vi "Serials.vi"() -> ()   [LabVIEW 2012]
panel:
  in  "ICImagingControl":refnum<k7>(container)
  out "Modelnames (hidden)":string[](array[string])
  out "Model Name":string
  out "Serials (hidden)":string[](array[string])
  in  "End Program":bool
  in  "Open & Snap":bool
  out "Serial":string
  in  "Devices":i32(listbox)
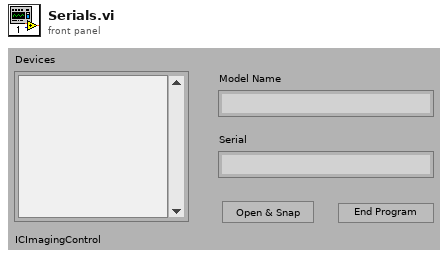
[diagram p1: front panel]
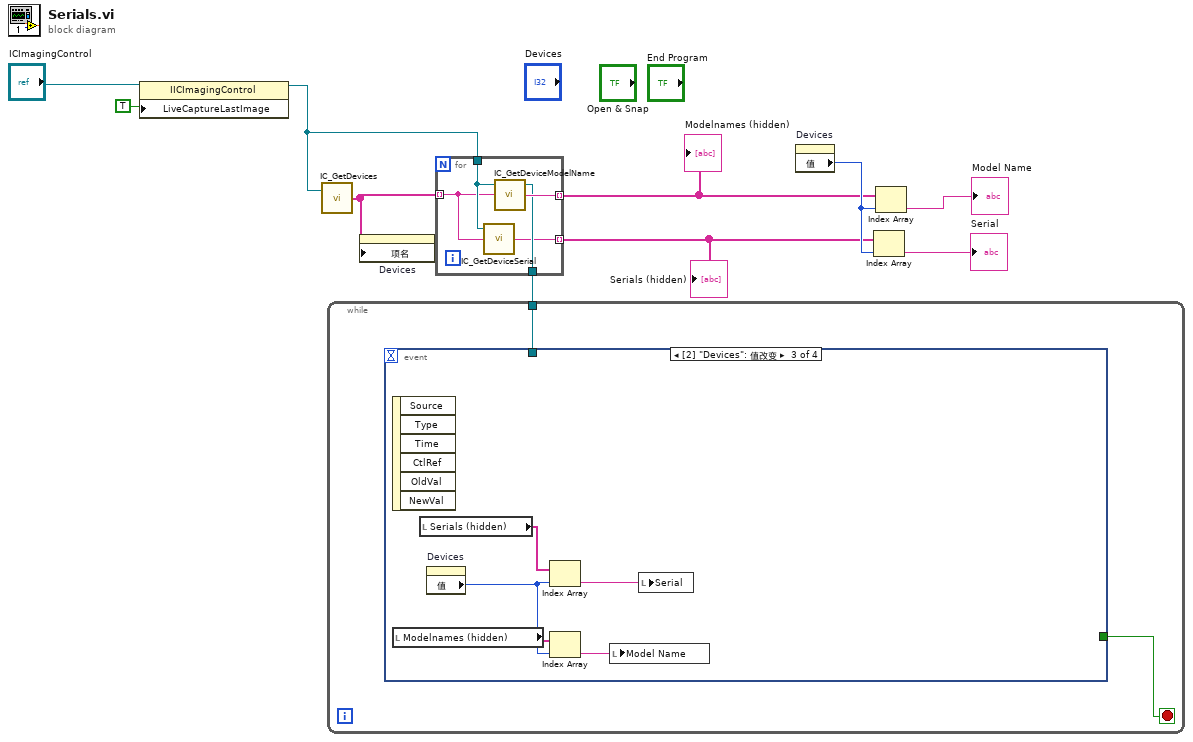
[diagram p0: block diagram]
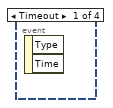
[diagram p2: hidden frame]
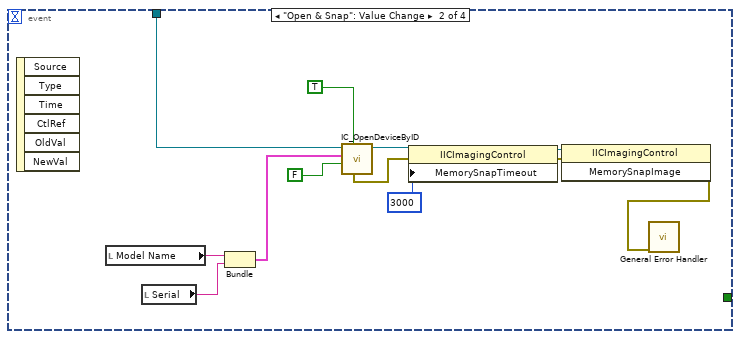
[diagram p3: hidden frame]
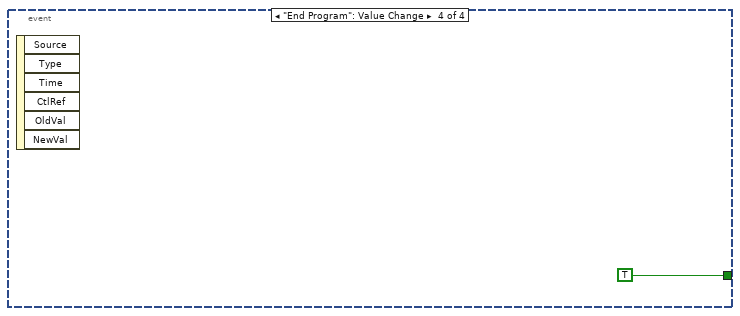
[diagram p4: hidden frame]
diagram:
  n1 = property class="IICImagingControl"(reference="ICImagingControl", "LiveCaptureLastImage"=TRUE) -> (reference out=w3:refnum<k7>)  [unwired: 1 in, 1 out]
  n2 = call <userlib>:"IC_GetDevices.vi"("ICImagingControl In"=w3) -> ("Devices"=w9:string[])  [unwired: 1 in, 2 out]
  n3 = property on="Devices" class="LstBox (严格)"("项名"=w9) -> ()  [unwired: 2 in, 2 out]
  n4 = for {
    tunnel: w9 -> [w12] mode=indexing
    tunnel: w3 -> [w13]
    tunnel: [w15] -> w7 mode=indexing
    tunnel: [w14] -> w10
    tunnel: [w11] -> w6 mode=indexing
    n5 = call <userlib>:"IC_GetDeviceSerial.vi"("Device"=w12, "ICImagingControl In"=w13) -> ("Serial"=w11:string)  [unwired: 1 in, 2 out]
    n6 = call "IC_GetDeviceModelName.vi"("Device"=w12, "ICImagingControl In"=w13) -> ("Basename"=w15:string, "ICImagingControl Out"=w14:refnum<k7>)  [unwired: 1 in, 1 out]
  }
  "Serials (hidden)" <- w6
  "Modelnames (hidden)" <- w7
  n7 = while {
    tunnel: w10 -> [w16]
    stop <- w17 stop-if-true
    n8 = event shown="[2] \"Devices\": 值改变" {
      selector: _ -> [_ _ _ _]
      dyn-events: _ -> [_ _ _ _]
      timeout: _ -> [_ _ _ _]
      tunnel: [_ _ _ TRUE] -> w17
      tunnel: w16 -> [_ w27 _ _]
      event Timeout {
        n9 = event-data() -> ()  [unwired: 1 in, 2 out]
      }
      event "Open & Snap": Value Change {
        n10 = event-data() -> ()  [unwired: 1 in, 6 out]
        n11 = local read "Model Name"() -> (w24:string)
        n12 = local read "Serial"() -> (w26:string)
        n13 = Bundle("Model Name"=w24, "Serial"=w26) -> (w25:cluster{"Model Name":string, "Serial":string})  [unwired: 1 in]
        n14 = call "IC_OpenDeviceByID.vi"("Color"=TRUE, "Live"=FALSE, "DeviceID"=w25, "ICImagingControl In"=w27) -> ("ICImagingControl Out"=w23:refnum<k7>, "Error Out"=w20:errorcluster)  [unwired: 2 in, 4 out]
        n15 = property class="IICImagingControl"(reference=w23, error in=w20, "MemorySnapTimeout"=3000) -> (reference out=w22:refnum<k7>, error out=w19:errorcluster)
        n16 = invoke class="IICImagingControl" method="MemorySnapImage"(reference=w22, error in=w19) -> (error out=w18:errorcluster)  [unwired: 1 in, 2 out]
        n17 = call <vilib>:"General Error Handler.vi"("error in (no error)"=w18) -> ()  [unwired: 10 in, 5 out]
      }
      event "Devices": Value Change {
        n18 = event-data() -> ()  [unwired: 1 in, 6 out]
        n19 = local read "Modelnames (hidden)"() -> (w31:string[])
        n20 = local read "Serials (hidden)"() -> (w34:string[])
        n21 = property on="Devices" class="LstBox (严格)"() -> ("值"=w32:i32)  [unwired: 2 in, 2 out]
        n22 = Index Array(array=w34, index=w32) -> (element=w33:string)
        n23 = Index Array(array=w31, index=w32) -> (element=w30:string)
        n24 = local write "Model Name"(w30) -> ()
        n25 = local write "Serial"(w33) -> ()
      }
      event "End Program": Value Change {
        n26 = event-data() -> ()  [unwired: 1 in, 6 out]
      }
    }
  }
  n27 = property on="Devices" class="LstBox (严格)"() -> ("值"=w8:i32)  [unwired: 2 in, 2 out]
  n28 = Index Array(array=w6, index=w8) -> (element=→"Serial":string)
  n29 = Index Array(array=w7, index=w8) -> (element=→"Model Name":string)
